vi "Control_PD_DAQ.vi"() -> ()   [LabVIEW 2012]
panel:
  out "Control":dbl
  in  "Entrada Deseada":dbl
  in  "c(k-2)":dbl
  in  "c(k-1)":dbl
  in  "stop":bool
  in  "d1":dbl=2.0
  in  "d2":dbl
  in  "d3":dbl
  in  "c1":dbl=0.0051
  in  "c2":dbl=1.025e-07
  in  "c3":dbl
  out "Error":dbl=1.651222908716221e-05
  in  "e(k-2)":dbl
  in  "e(k-1)":dbl
  out "Salida y(k)":dbl(graph)=2.000016512205615
  # "CONTROLADOR"
  # "Z  +"
  # "Z^2  +"
  # "Gp(z) = --------------------------------------------------------"
  # "Z^2  +"
  # "Z  +"
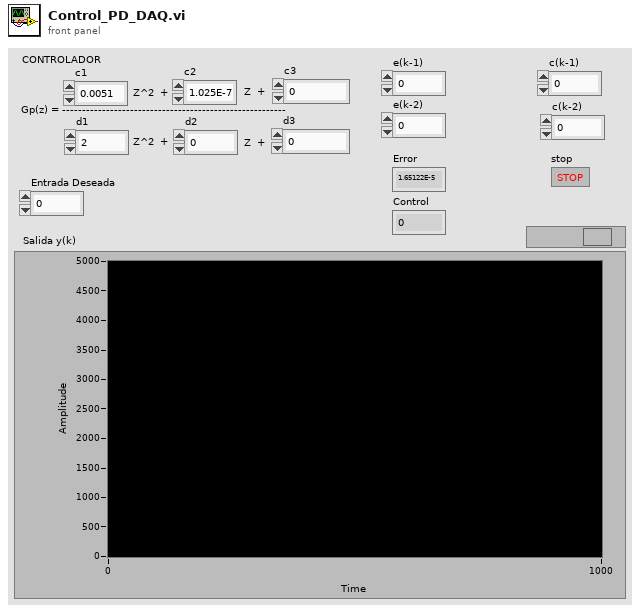
[diagram p1: front panel]
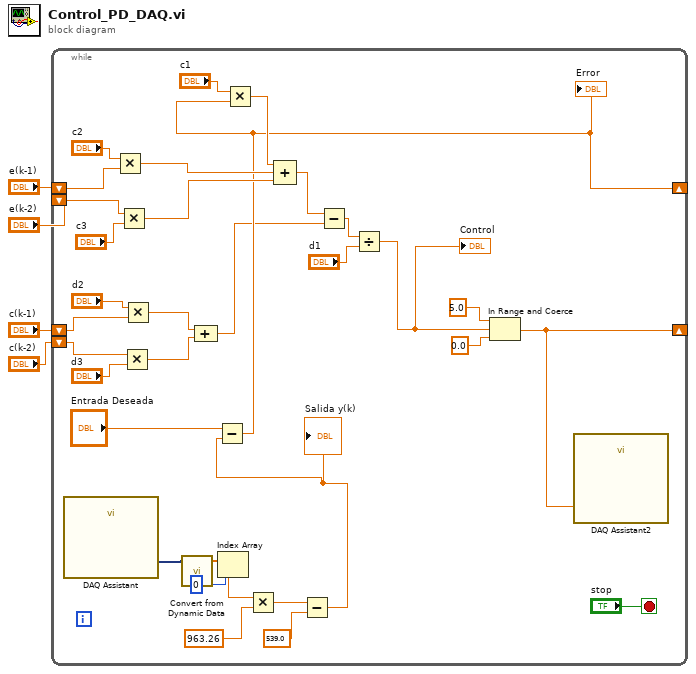
[diagram p0: block diagram]
diagram:
  n1 = while {
    shift-right: [w29] -> _
    shift-left: "e(k-1)" -> [w37]
    shift-left: "e(k-2)" -> [w36]
    shift-right: [w10] -> _
    shift-left: "c(k-1)" -> [w19]
    shift-left: "c(k-2)" -> [w18]
    stop <- "stop" stop-if-true
    n2 = call "DAQ Assistant"() -> ("data"=w11:dynamicdata)  [unwired: 17 in, 2 out]
    n3 = Multiply(x="c2", y=w37) -> (x*y=w35:dbl)
    n4 = Multiply(x=w36, y="c3") -> (x*y=w34:dbl)
    n5 = Multiply(x=w18, y="d3") -> (x*y=w22:dbl)
    n6 = Multiply(x="d2", y=w19) -> (x*y=w23:dbl)
    n7 = call "Convert from Dynamic Data"("Dynamic Data Type"=w11) -> ("Array"=w15:dbl[])  [unwired: 3 in]
    n8 = Compound Arithmetic op=ADD(w23, w22) -> (w21:dbl)
    n9 = Index Array(array=w15, index=0) -> (element=w6:dbl)
    n10 = Multiply(x=w6, y=963.26) -> (x*y=w8:dbl)
    n11 = Subtract(x=w8, y=539.0) -> (x-y=w5:dbl)
    "Salida y(k)" <- w5
    n12 = Subtract(x="Entrada Deseada", y=w5) -> (x-y=w29:dbl)
    "Error" <- w29
    n13 = Multiply(x="c1", y=w29) -> (x*y=w31:dbl)
    n14 = Compound Arithmetic op=ADD(w31, w35, w34) -> (w33:dbl)
    n15 = Subtract(x=w33, y=w21) -> (x-y=w32:dbl)
    n16 = Divide(x=w32, y="d1") -> (x/y=w13:dbl)
    "Control" <- w13
    n17 = In Range and Coerce(upper limit=5.0, x=w13, lower limit=0.0) -> (coerced(x)=w10:dbl)  [unwired: 1 out]
    n18 = call "DAQ Assistant2"("data"=w10) -> ()  [unwired: 17 in, 2 out]
  }
